vi "Read FIFOs and Queue.vi"(0 "FPGA VI Reference":T1, 5 "Data Size":u32, 7 "# Elements to Read":u32, 9 "# Data Sets To Read":u32, 11 "error in (no error)":errorcluster, 12 "Sync Guard Data":fxp<+/-,38,12>[](array[numeric])=[888.2284999489784, 399.7682446986437, -617.0920498371124] format="%.9g") -> (3 "Read Mismatch":bool, 4 "Refnum out":T1, 6 "Elements Remaining":u32, 8 "Data Unfiltered":fxp<+/-,38,12>[][](array[numeric]), 10 "DataFiltered":fxp<+/-,38,12>[][](array[numeric]), 15 "error out":errorcluster)   [LabVIEW 2020]
doc: "Author: Scott Hannahs <sth@magnet.fsu.edu>\nCopyright 2018 Florida State University, All rights reserved."
uses:
  RT Controls/FPGA SCH Digitizer Ref.ctl
  <vilib>/Utility/error.llb/Error Cluster From Error Code.vi
  <vilib>/rvi/errors/niLvFpgaAdjustHostInterfaceError.vi
  <vilib>/rvi/interface/nirviMethod/nirviMethod.xnode
  <vilib>/FPGAPlugInAG/Dynamic/niLvFpga_ReadFifo_Dynamic.vi
  <vilib>/rvi/errors/niLvFpgaMergeErrorWithErrorCode.vi
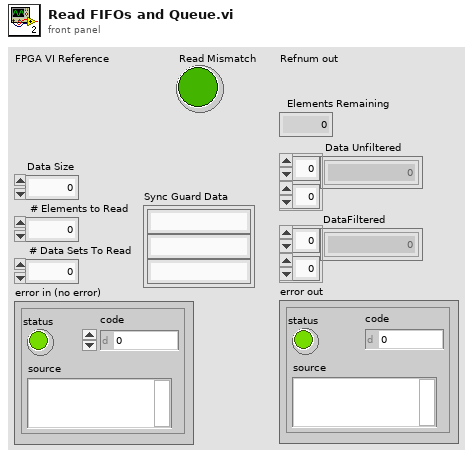
[diagram p1: front panel]
types:
  T1 = typedef "FPGA SCH Digitizer Ref.ctl" = refnum<k20>
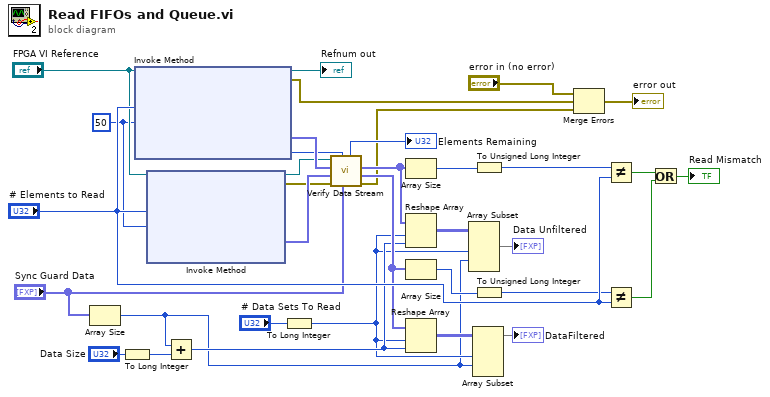
[diagram p0: block diagram]
diagram:
  w17 = 50 ("Timeout (ms)")
  n1 = Array Size(array="Sync Guard Data") -> (size(s)=w1:i32)
  n2 = To Long Integer(number="Data Size") -> (32bit integer=w5:i32)
  n3 = xnode "Invoke Method"("FPGA VI Reference In"="FPGA VI Reference", "Number of Elements"="# Elements to Read", "Timeout (ms)"=w17) -> ("FPGA VI Reference Out"=→"Refnum out":T1, "error out"=w19:errorcluster, "Data"=w14:fxp<+/-,38,12>[], "Elements Remaining"=w11:u32)  [unwired: 1 in]
  n4 = xnode "Invoke Method"("FPGA VI Reference In"="FPGA VI Reference", "Number of Elements"="# Elements to Read", "Timeout (ms)"=w17) -> ("FPGA VI Reference Out"=w8:T1, "error out"=w10:errorcluster, "Data"=w16:fxp<+/-,38,12>[])  [unwired: 1 in, 1 out]
  n5 = Add(x=w1, y=w5) -> (x+y=w7:i32)
  n6 = To Long Integer(number="# Data Sets To Read") -> (32bit integer=w2:i32)
  n7 = call "Verify Data Stream.vi"("Sync Guard Data"="Sync Guard Data", "Elements Remaining In"=w11, "error in (no error)"=w10, "DataFiltered In"=w16, "Data Unfiltered In"=w14, "FPGA VI Reference"=w8) -> ("error out"=w9:errorcluster, "DataFiltered Out"=w15:fxp<+/-,38,12>[], "Data Unfiltered Out"=w13:fxp<+/-,38,12>[], "Elements Remaining"=→"Elements Remaining":u32)  [unwired: 1 in, 1 out]
  n8 = Array Size(array=w13) -> (size(s)=w23:i32)
  n9 = Reshape Array(w13, w2, w7) -> (w30:fxp<+/-,38,12>[][])
  n10 = Array Size(array=w15) -> (size(s)=w21:i32)
  n11 = Reshape Array(w15, w2, w7) -> (w27:fxp<+/-,38,12>[][])
  n12 = Array Subset(array=w30, length (row)=w2, index (col)=w1) -> (→"Data Unfiltered":fxp<+/-,38,12>[][])  [unwired: 2 in]
  n13 = Array Subset(array=w27, length (row)=w2, index (col)=w1) -> (→"DataFiltered":fxp<+/-,38,12>[][])  [unwired: 2 in]
  n14 = To Unsigned Long Integer(number=w23) -> (unsigned 32bit integer=w29:u32)
  n15 = To Unsigned Long Integer(number=w21) -> (unsigned 32bit integer=w28:u32)
  n16 = Merge Errors("error in (no error)", w19, w9) -> (→"error out":errorcluster)
  n17 = Not Equal?(x=w29, y="# Elements to Read") -> (x != y?=w25:bool)
  n18 = Not Equal?(x=w28, y="# Elements to Read") -> (x != y?=w22:bool)
  n19 = Or(x=w25, y=w22) -> (x .or. y?=→"Read Mismatch":bool)
